vi "FileSzieDiffercneCheck.vi"() -> ()   [LabVIEW 2020]
panel:
  out "Array":path[](array[path])
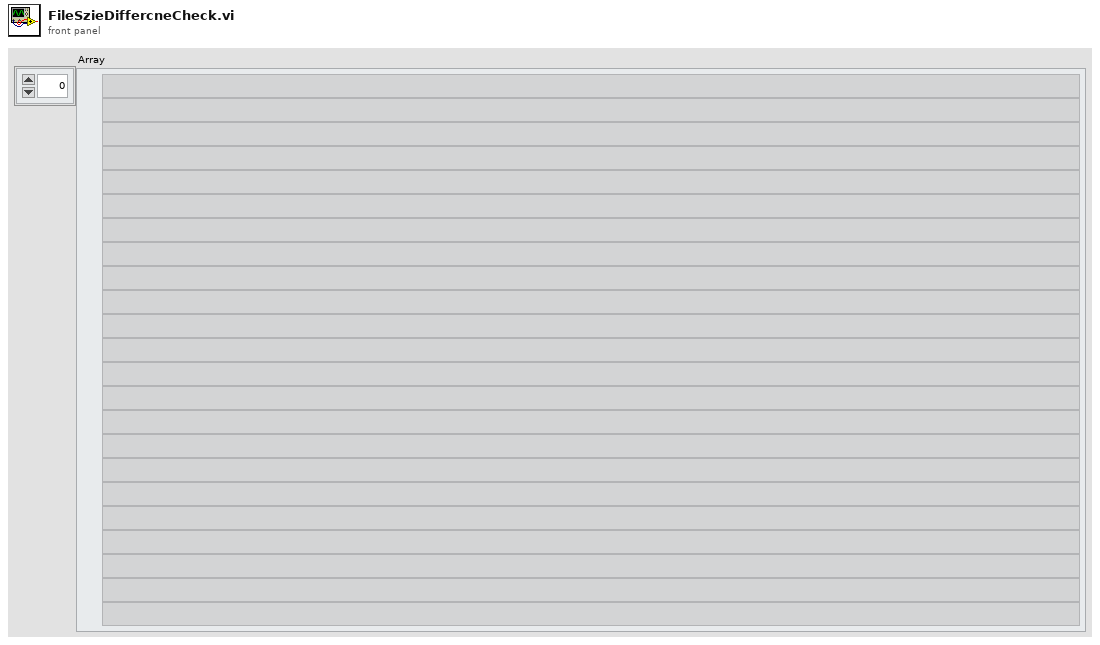
[diagram p1: front panel]
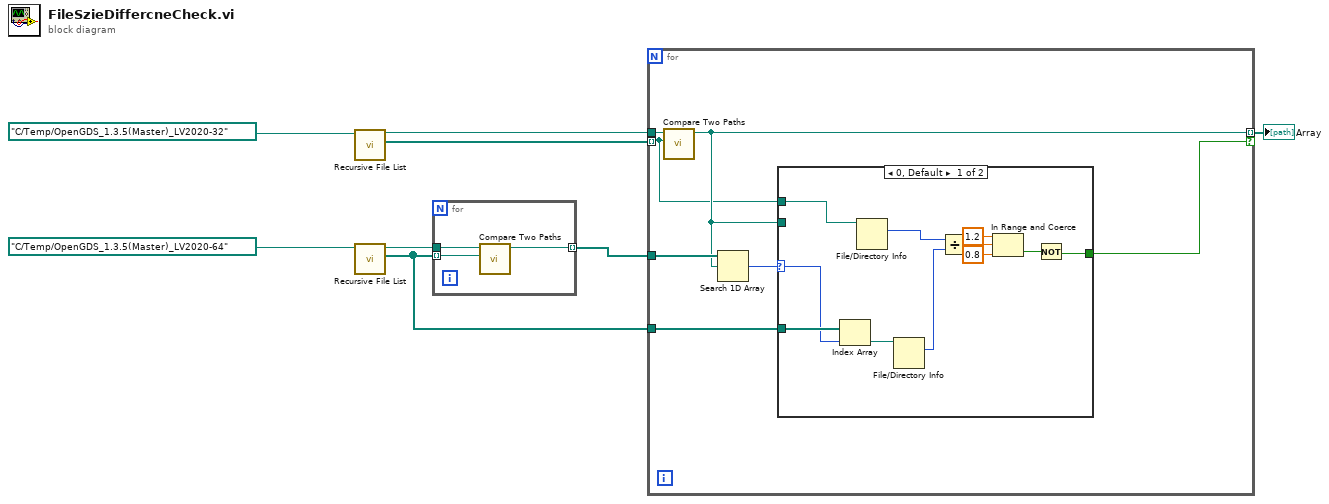
[diagram p0: block diagram]
diagram:
  n1 = call <vilib>:"Recursive File List.vi"("Folder Path"=path "C:/Temp/OpenGDS_1.3.5(Master)_LV2020-32") -> ("All Files in Dir"=w6:path[], "dup Folder Path"=w5:path)  [unwired: 6 in, 3 out]
  n2 = call <vilib>:"Recursive File List.vi"("Folder Path"=path "C:/Temp/OpenGDS_1.3.5(Master)_LV2020-64") -> ("All Files in Dir"=w1:path[], "dup Folder Path"=w4:path)  [unwired: 6 in, 3 out]
  n3 = for {
    tunnel: w1 -> [w11] mode=indexing
    tunnel: w4 -> [w10]
    tunnel: [w9] -> w3 mode=indexing
    n4 = call <vilib>:"Compare Two Paths.vi"("Path 2"=w11, "Path 1"=w10) -> ("Relative Path from 1 to 2"=w9:path)  [unwired: 6 in, 3 out]
  }
  n5 = for {
    tunnel: w6 -> [w12] mode=indexing
    tunnel: w3 -> [w16]
    tunnel: w5 -> [w18]
    tunnel: [w15] -> w2 mode=indexing if=w14
    tunnel: w1 -> [w13]
    n6 = call <vilib>:"Compare Two Paths.vi"("Path 2"=w12, "Path 1"=w18) -> ("Relative Path from 1 to 2"=w15:path)  [unwired: 6 in, 3 out]
    n7 = Search 1D Array(1D array=w16, element=w15) -> (index of element=w17:i32)  [unwired: 1 in]
    n8 = case shown="0, Default" w17 {
      selector: w17 -> [w28 _]
      tunnel: w15 -> [_ _]
      tunnel: w13 -> [w29 _]
      tunnel: [w20 _] -> w14
      tunnel: w12 -> [w19 _]
      frame 0, Default {
        n9 = Index Array(array=w29, index=w28) -> (element=w27:path)
        n10 = File/Directory Info(path=w19) -> (size=w26:i64)  [unwired: 1 in, 6 out]
        n11 = File/Directory Info(path=w27) -> (size=w25:i64)  [unwired: 1 in, 6 out]
        n12 = Divide(x=w26, y=w25) -> (x/y=w24:dbl)
        n13 = In Range and Coerce(upper limit=1.2, x=w24, lower limit=0.8) -> (In Range?=w21:bool)  [unwired: 1 out]
        n14 = Not(x=w21) -> (.not. x?=w20:bool)
      }
      frame -1 {
      }
    }
  }
  "Array" <- w2
